vi "Cannon Problem Fix.vi"(1 "Cannon Global Data Modified":T2, 2 "Cannon Global Data Original":T2) -> (0 "Cannon Global Data New":T2)   [LabVIEW 2013]
uses:
  <vilib>/Rock Robotics/WPI/Solenoid/WPI_SolenoidValue.ctl
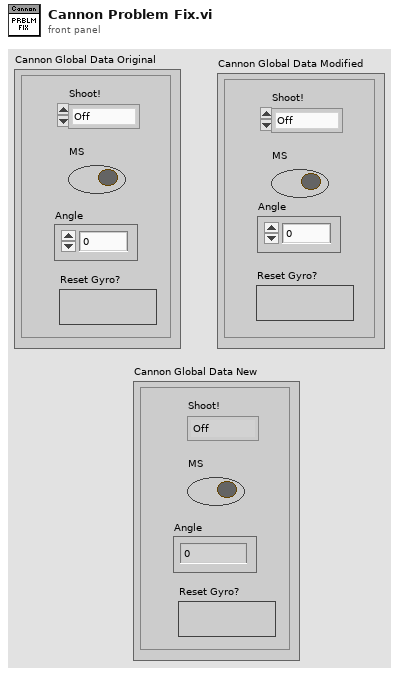
[diagram p1: front panel]
types:
  T1 = typedef "WPI_SolenoidValue.ctl" = enum16{"Off", "On", "Forward", "Reverse"}
  T2 = cluster{"MS":bool, "Shoot!":T1, "Angle":dbl, "Reset Gyro?":bool}
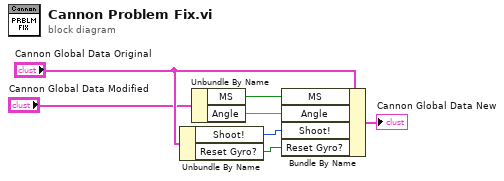
[diagram p0: block diagram]
diagram:
  n1 = Unbundle By Name("Cannon Global Data Original") -> ("Shoot!"=w1:T1, "Reset Gyro?"=w3:bool)
  n2 = Unbundle By Name("Cannon Global Data Modified") -> ("MS"=w4:bool, "Angle"=w2:dbl)
  n3 = Bundle By Name(cluster="Cannon Global Data Original", "MS"=w4, "Angle"=w2, "Shoot!"=w1, "Reset Gyro?"=w3) -> (→"Cannon Global Data New":T2)
